vi "Actor Core.vi"(8 "error in":errorcluster, 11 "Driver in":refnum<class "Driver.lvclass">) -> (0 "error out":errorcluster, 3 "Actor out":refnum<class "Actor.lvclass">)   [LabVIEW 2013, in "Driver.lvlib" / "Driver.lvclass"]
doc: "(<B>Filename</B>: Actor Framework.lvlib:Actor.lvclass:Actor Core.vi)\n\nReceives messages to the actor, reacts to them, and initiates any error handling that may shut the actor down.\n\nDescendant classes may override this VI to append parallel tasks for the actor to complete while it handles messages. Overrides use the Call Parent Method node."
uses:
  Driver.lvclass
  <vilib>/ActorFramework/Actor/Actor.lvclass
  <vilib>/ActorFramework/Actor/Actor.lvclass/Actor.ctl
  <vilib>/ActorFramework/Message Enqueuer/Message Enqueuer.lvclass/Message Enqueuer.ctl
  Driver.lvclass/Driver.ctl
  XBoxController/XBoxController.lvclass
  VirtualRobot/Systems/XBoxController-V.lvclass
  <vilib>/ActorFramework/Message Enqueuer/Init from Existing Queue.vi
  <vilib>/ActorFramework/Message Enqueuer/Message Enqueuer.lvclass
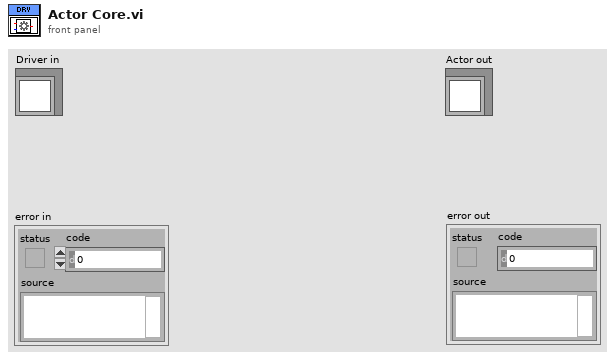
[diagram p1: front panel]
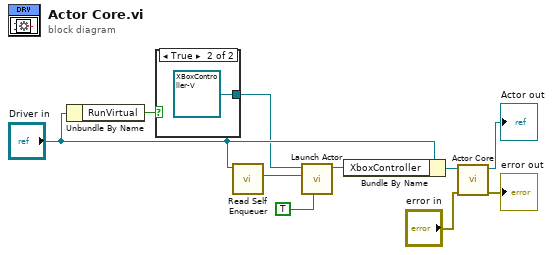
[diagram p0: block diagram]
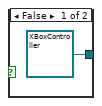
[diagram p2: hidden frame]
diagram:
  n1 = Unbundle By Name("Driver in") -> ("RunVirtual"=w2:bool)
  n2 = case shown="True" w2 {
    tunnel: [refnum<class "XBoxController.lvclass"> refnum ("XBoxController.lvlib:XBoxController.lvclass") refnum<class "XBoxController-V.lvclass"> refnum ("VirtualRobot.lvlib:XBoxController-V.lvlib:XBoxController-V.lvclass")] -> w1
    frame False {
    }
    frame True {
    }
  }
  n3 = call <vilib>:"Read Self Enqueuer.vi"("Actor"="Driver in") -> ("Self Enqueuer"=w7:refnum<class "Message Enqueuer.lvclass">)  [unwired: 10 in]
  n4 = call <vilib>:"Launch Actor.vi"("Open Actor Core front panel? (F)"=TRUE, "Actor-to-Caller Enqueuer"=w7, "Actor"=w1) -> ("Caller-To-Actor Enqueuer"=w5:refnum<class "Message Enqueuer.lvclass">)  [unwired: 7 in, 1 out]
  n5 = Bundle By Name(cluster="Driver in", "XboxController"=w5) -> (w6:refnum<class "Driver.lvclass">)
  n6 = call-parent "Actor Core.vi"("error in"="error in", "Actor in"=w6) -> ("error out"=→"error out":errorcluster, "Actor out"=→"Actor out":refnum<class "Actor.lvclass">)  [unwired: 8 in]
